vi "Test 03.vi"() -> ()   [LabVIEW 2021]
uses:
  <vilib>/Platform/TimedLoop/XDataNode/timing_clust.ctl
  <vilib>/Platform/TimedLoop/XDataNode/nitl_modes.ctl
  <vilib>/Platform/TimedLoop/XDataNode/wakeup.ctl
  <vilib>/MakerHub/LINX/Public/Utilities/Open Serial.vi
  <vilib>/Utility/file.llb/Write Delimited Spreadsheet (DBL).vi
  <vilib>/platform/TimedLoop/XDataNode/XDataNode.xnode
  <vilib>/Platform/TimedLoop/XDataNode/XDNodeRunTimeDep.lvlib
  <vilib>/MakerHub/LINX/LMH-LINX.lvlib
panel:
  out "theta offset":dbl
  out "dt":dbl
  out "Overrun":bool
  in  "Serial Port":refnum<visa-resource-name>
  in  "Stop Button":bool
  out "theta":dbl(graph)=0.10008950000019468
  in  "Motor command":dbl
  in  "Enable friction compensation":bool=TRUE
  in  "Friction compensation":dbl=0.07
  in  "Reset":bool
  in  "Kp":dbl=15.0
  out "omega":dbl(graph)
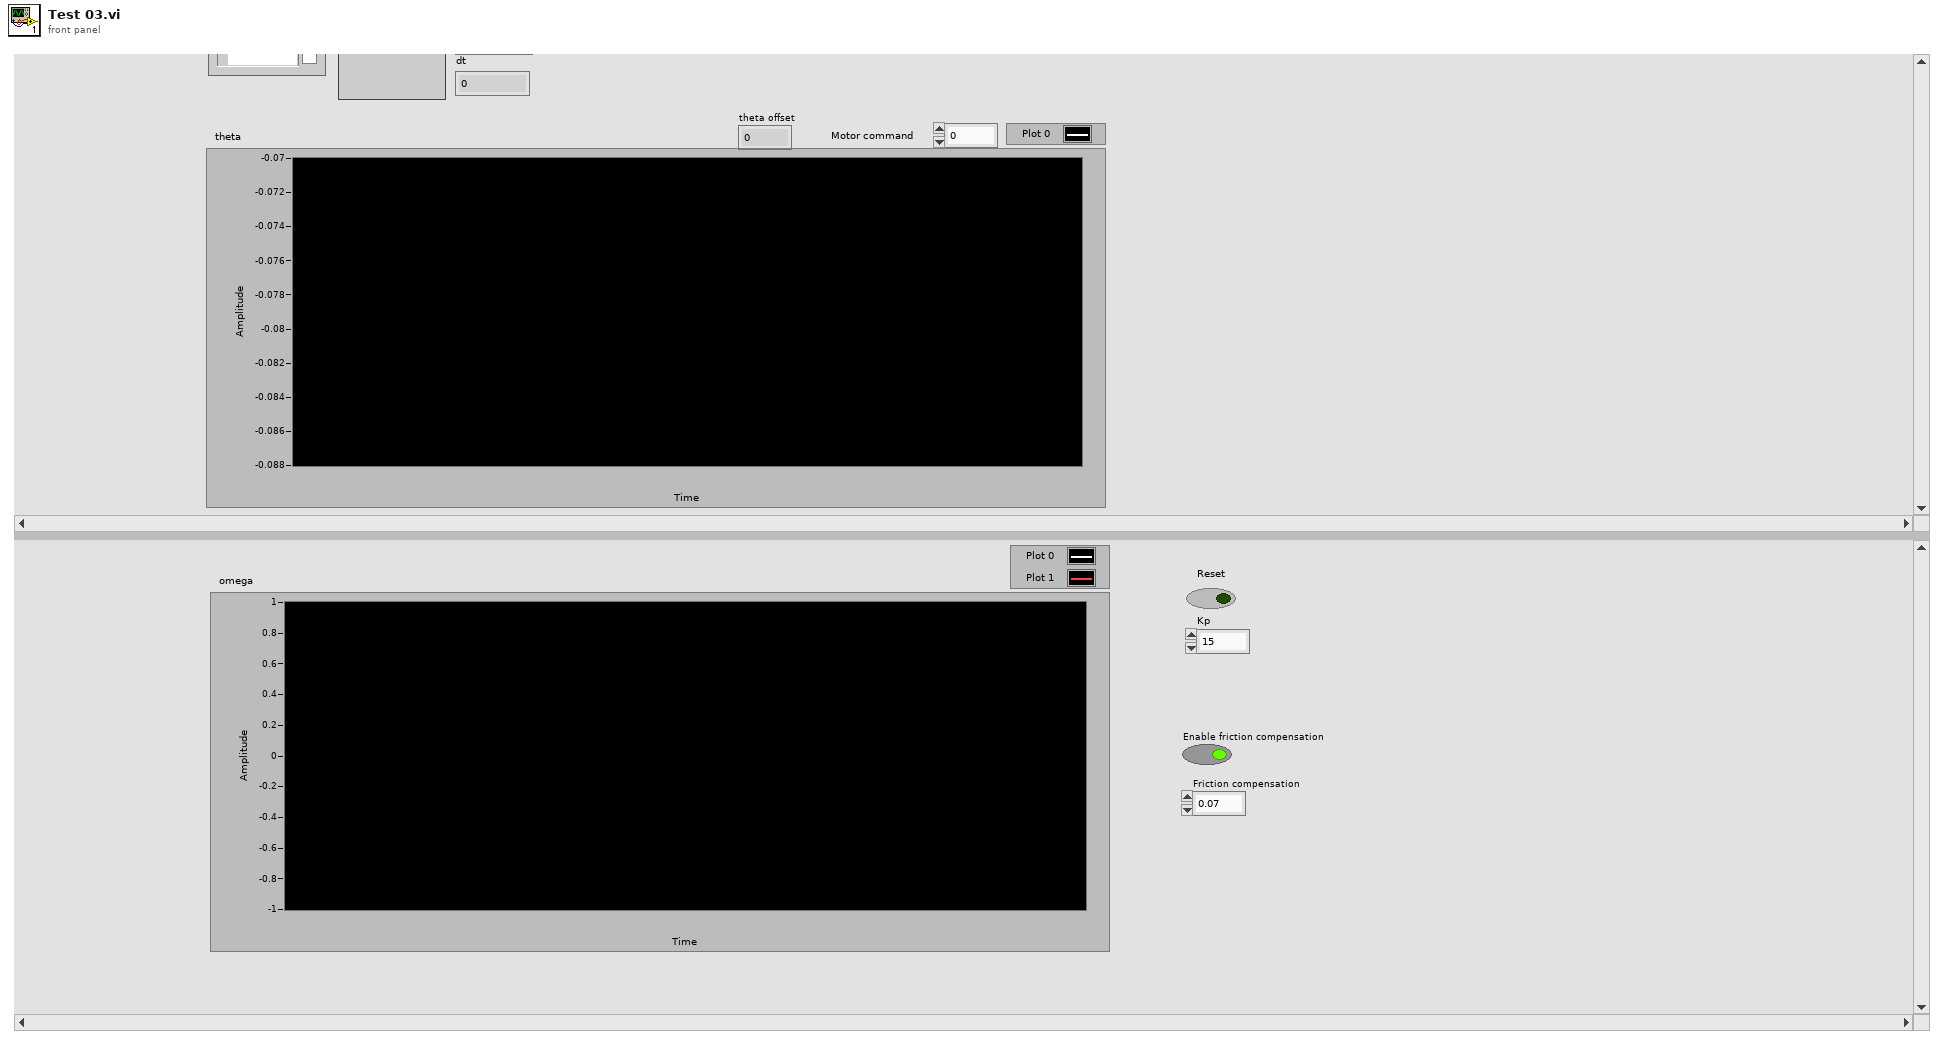
[diagram p1: front panel]
types:
  T1 = typedef "XDNodeRunTimeDep.lvlib/timing_clust.ctl" = cluster{"Expected End [f-1]":u64, "Actual End [f-1]":u64, "Finished Late? [f-1]":bool, "Expected End [i-1]":u64, "Actual End [i-1]":u64, "Finished Late? [i-1]":bool, "Expected Start [i]":u64, "Actual Start [i]":u64, "Expected Start [f]":u64, "Actual Start [f]":u64, "Source Name":string, "Structure Name":string, "Period":i64, "Deadline":i64, "Offset":i64, "Start":i64, "Priority":i32, "Timeout":i32, "Mode":T2, "Wakeup Reason":T3, "Error":errorcluster, "Source Type":string, "Secondary Source Type":string, "Global End Time":u64, "Global Start Time":u64, "Frame Duration":u64, "Iteration Duration":u64, "Assigned CPU":i32, "I/O Scan Engine Mode":u32}
  T2 = typedef "XDNodeRunTimeDep.lvlib/nitl_modes.ctl" = enum32{"No Change", "Process missed periods, maintain original phase", "Discard missed periods, maintain original phase", "Process missed periods, ignore original phase", "Discard missed periods, ignore original phase"}
  T3 = typedef "XDNodeRunTimeDep.lvlib/wakeup.ctl" = enum32{"Normal", "Aborted", "Asynchronous wakeup", "Timing source error", "Timed loop error", "Timeout"}
  T4 = typedef "LMH-LINX.lvlib/LINX Ref.ctl" = cluster{"IO":T5, "Interface":T6, "LINX Device Config":T7}
  T5 = typedef "LMH-LINX.lvlib/Platform.ctl" = enum16{"Remote", "Local"}
  T6 = typedef "LMH-LINX.lvlib/Interface.ctl" = enum16{"Serial", "TCP"}
  T7 = typedef "LMH-LINX.lvlib/Device.lvlib/LINX Device Config.ctl" = cluster{"Interface":T6, "COM Port":refnum<visa-resource-name>, "TCP Configuration":T8, "Device Family":u8, "Device ID":u8, "Device Name":string, "TCP Ref":refnum<k5>, "Channels":T9}
  T8 = typedef "LMH-LINX.lvlib/Device.lvlib/TCP Config.ctl" = cluster{"IP Address":string, "Port":u16}
  T9 = typedef "LMH-LINX.lvlib/Channels.ctl" = cluster{"DI":u8[], "DO":u8[], "AI":u8[], "AO":u8[], "PWM":u8[], "QE":u8[], "UART":u8[], "I2C 2":u8[], "SPI":u8[], "CAN":u8[], "Servo":u8[], "AI Ref (V)":dbl, "AI Resolution (Bits)":u8, "AO Ref (V)":dbl, "AO Resolution (Bits)":u8}
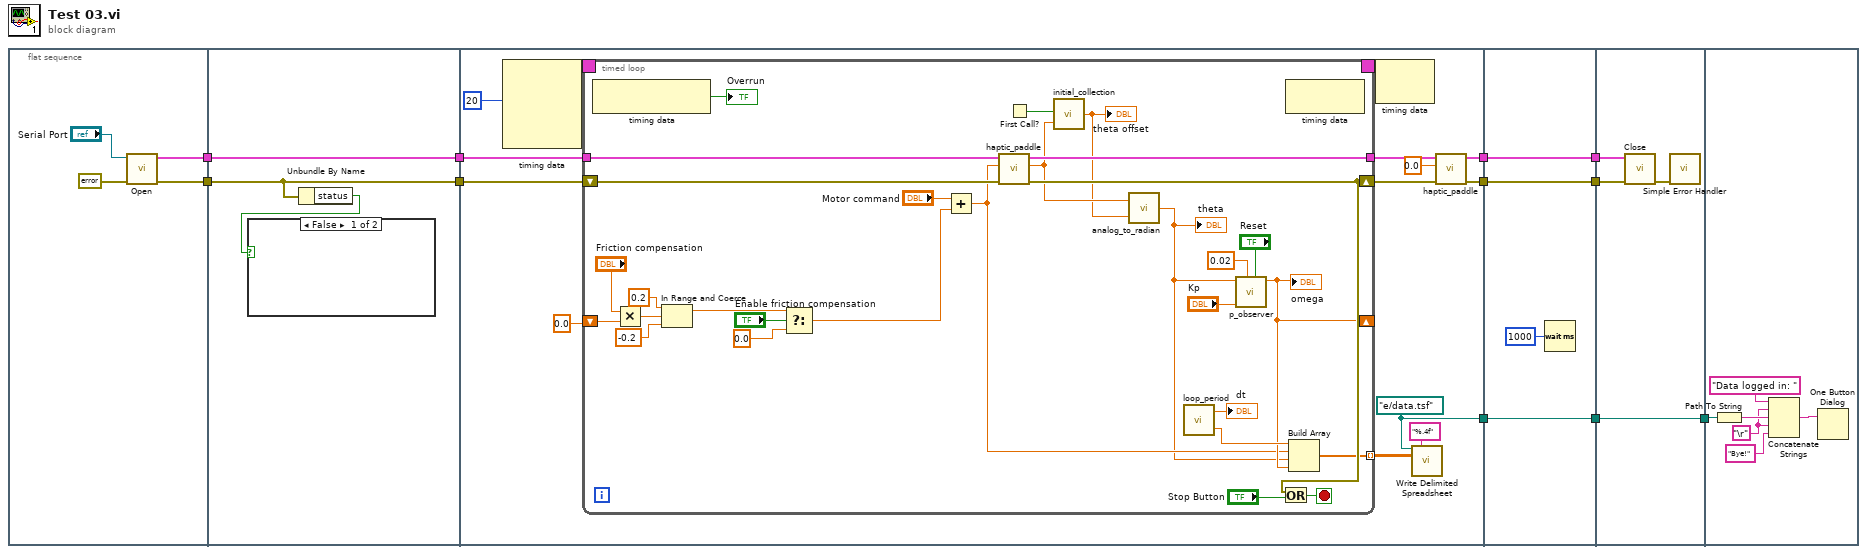
[diagram p0: block diagram]
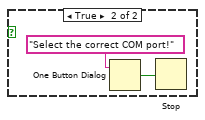
[diagram p2: hidden frame]
diagram:
  n1 = flat-sequence {
    tunnel: [w13] -> w7
    tunnel: [w12] -> w5
    tunnel: w7 -> [w18]
    tunnel: [w18] -> w6
    tunnel: w5 -> [w17]
    tunnel: [w17] -> w4
    tunnel: [w29] -> w10
    tunnel: [w28] -> w8
    tunnel: w6 -> [w27]
    tunnel: w4 -> [w26]
    tunnel: [w22] -> w3
    tunnel: [w73] -> w11
    tunnel: w10 -> [w73]
    tunnel: [w72] -> w9
    tunnel: w8 -> [w72]
    tunnel: w3 -> [w71]
    tunnel: [w71] -> w2
    tunnel: w11 -> [w77]
    tunnel: w9 -> [w76]
    tunnel: w2 -> [w75]
    tunnel: [w75] -> w1
    tunnel: w1 -> [w84]
    frame #0 {
      n2 = call-poly <vilib>:"Open.vi"("Error In"=errorcluster {"status"=FALSE, "code"=0, "source"=""}, "Serial Port"="Serial Port") -> ("Error Out"=w12:errorcluster, "LINX Resource"=w13:T4)  [unwired: 7 in, 1 out]
    }
    frame #1 {
      n3 = Unbundle By Name(w17) -> ("status"=w16:bool)
      n4 = case shown="False" w16 {
        frame False {
        }
        frame True {
          n5 = One Button Dialog(message="Select the correct COM port!") -> (true=w19:bool)  [unwired: 1 in]
          n6 = Stop(stop? (T)=w19) -> ()
        }
      }
    }
    frame #2 {
      w22 = path "e:/data.tsf" ("file path (dialog if empty)")
      n7 = node-c288(i64 20 ("Period")) -> (w34:T1)  [unwired: 3 in]
      n8 = timed-loop {
        tunnel: w27 -> [w59]
        tunnel: [w61] -> w31
        shift-right: [w60] -> w30
        shift-left: w26 -> [w58]
        timing: w34 -> [_]
        timing-out: [_] -> w33
        tunnel: [w57] -> w24 mode=indexing
        shift-right: [w50] -> _
        shift-left: 0.0 ("y_dot") -> [w49]
        stop <- w63 stop-if-true
        n9 = node-c288() -> (→"Overrun":bool)  [unwired: 1 in]
        n10 = Multiply(x="Friction compensation", y=w49) -> (x*y=w45:dbl)
        n11 = In Range and Coerce(upper limit=0.2, x=w45, lower limit=-0.2) -> (coerced(x)=w42:dbl)  [unwired: 1 out]
        n12 = Select(t=w42, s="Enable friction compensation", f=0.0) -> (s? t:f=w41:dbl)
        n13 = Add(x="Motor command", y=w41) -> (x+y=w46:dbl)
        n14 = call "haptic_paddle.vi"("Error In"=w58, "PWM Input"=w46, "LINX Resource In"=w59) -> ("Error Out"=w60:errorcluster, "Angular Output"=w37:dbl, "LINX Resource Out"=w61:T4)  [unwired: 6 in]
        n15 = First Call?() -> (First Call?: T/F=w38:bool)
        n16 = call "initial_collection.vi"("Input"=w37, "Flag"=w38) -> ("Ouput"=w35:dbl)
        "theta offset" <- w35
        n17 = call "analog_to_radian.vi"("Offset"=w35, "Analog signal"=w37) -> ("Radians"=w36:dbl)
        "theta" <- w36
        n18 = call "loop_period.vi"() -> ("t"=w51:dbl, "dt"=→"dt":dbl)  [unwired: 3 in]
        n19 = call "p_observer.vi"("y"=w36, "Kp"="Kp", "dt"=0.02, "Reset"="Reset") -> ("y_dot"=w50:dbl)  [unwired: 6 in]
        "omega" <- w50
        n20 = Or(x=w60, y="Stop Button") -> (x .or. y?=w63:bool)
        n21 = node-c288() -> ()  [unwired: 1 in, 1 out]
        n22 = Build Array(w51, w46, w36, w50) -> (w57:dbl[])
      }
      n23 = node-c288(w33) -> ()  [unwired: 1 out]
      n24 = call-poly <vilib>:"Write Delimited Spreadsheet.vi"("file path (dialog if empty)"=w22, "format (%.3f)"="%.4f", "2D data"=w24) -> ()  [unwired: 11 in, 2 out]
      n25 = call "haptic_paddle.vi"("Error In"=w30, "PWM Input"=0.0, "LINX Resource In"=w31) -> ("Error Out"=w28:errorcluster, "LINX Resource Out"=w29:T4)  [unwired: 6 in, 1 out]
    }
    frame #3 {
      n26 = Wait (ms)(milliseconds to wait=u32 1000) -> ()  [unwired: 1 out]
    }
    frame #4 {
      n27 = call <vilib>:"Close.vi"("Error In"=w76, "LINX Resource"=w77) -> ("Error Out"=w78:errorcluster)  [unwired: 9 in]
      n28 = call <vilib>:"Simple Error Handler.vi"("error in (no error)"=w78) -> ()  [unwired: 4 in, 5 out]
    }
    frame #5 {
      w79 = "\r"
      n29 = Path To String(path=w84) -> (string=w83:string)
      n30 = Concatenate Strings("Data logged in: " ("message"), w79, w83, w79, "Bye!" ("string")) -> (w81:string)
      n31 = One Button Dialog(message=w81) -> ()  [unwired: 1 in, 1 out]
    }
  }
